vi "Run.vi"(7 "Team Index":i32, 8 "Column":i32, 9 "Row":i32, 10 "View":i32[](array[numeric]) caption="View (Team Index, -1: empty)", 11 "DNatt In":refnum<class "DNatt.lvclass">) -> (0 "Replicated":refnum<class "Square.lvclass">, 1 "Direction":T1, 2 "Action":T2, 3 "DNatt Out":refnum<class "Square.lvclass">)   [LabVIEW 2015, in "DNatt.lvclass"]
uses:
  DNatt.lvclass
  Square/Square.lvclass
  Type Defs/Action Enum.ctl
  Type Defs/Direction Enum.ctl
  DNatt.lvclass/DNatt.ctl
  Common/Position.ctl
  SubVIs/Read-Only Globals.vi
  SubVIs/Globals (private).vi
  Common/Common.lvlib
  Type Defs/SB Type Defs.lvlib
panel:
  # "NW\nN\nNE\nE\nSE\nS\nSW\nW"
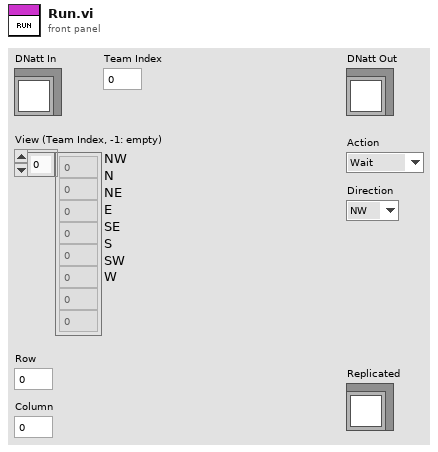
[diagram p1: front panel]
types:
  T1 = typedef "SB Type Defs.lvlib/Direction Enum.ctl" = enum16{"NW", "N", "NE", "E", "SE", "S", "SW", "W"}
  T2 = typedef "SB Type Defs.lvlib/Action Enum.ctl" = enum16{"Wait", "Move", "Attack", "Replicate"}
  T3 = typedef "Common.lvlib/Map DVR.ctl" = refnum<data-value>
  T4 = typedef "Common.lvlib/Position.ctl" = cluster{"Column":i32, "Row":i32}
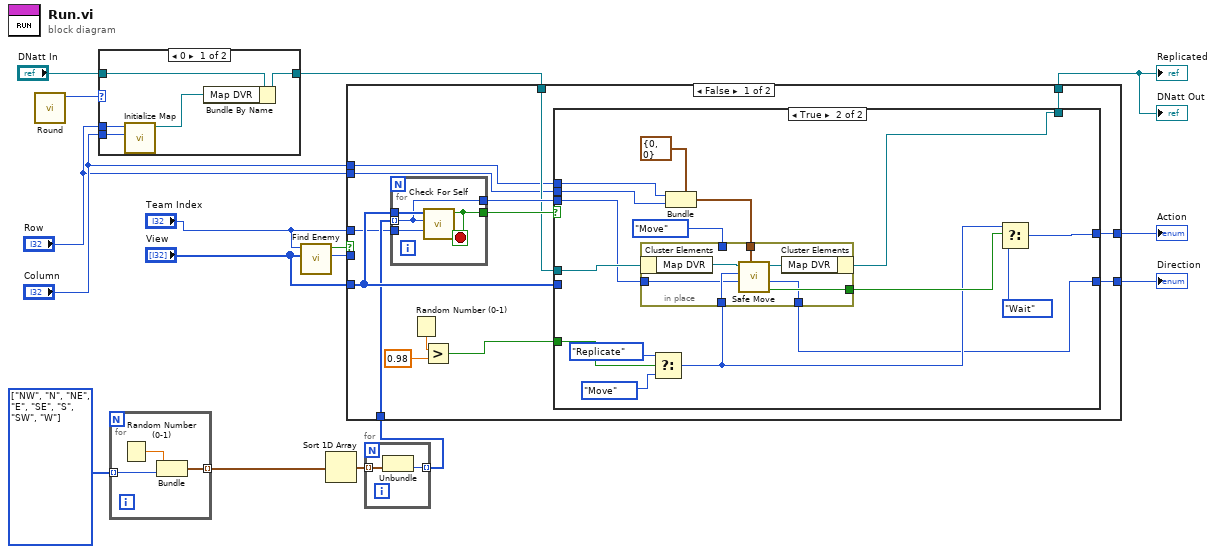
[diagram p0: block diagram]
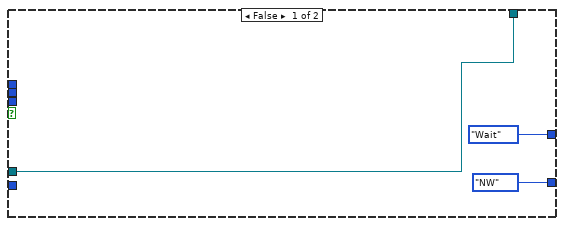
[diagram p3: hidden frame]
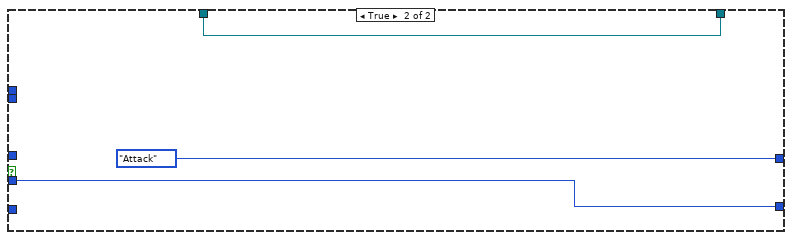
[diagram p4: hidden frame]
diagram:
  w11 = T1[] [enum."NW", enum."N", enum."NE", enum."E", enum."SE", enum."S", enum."SW", enum."W"] items=["NW", "N", "NE", "E", "SE", "S", "SW", "W"]
  n1 = call "Round.vi"() -> ("Round"=w6:i32)  [unwired: 11 in]
  n2 = case shown="0" w6 {
    tunnel: "DNatt In" -> [w19 w22]
    tunnel: [w18 w22] -> w5
    tunnel: "Row" -> [w21 _]
    tunnel: "Column" -> [w20 _]
    frame 0 {
      n3 = call "Initialize Map.vi"("Column"=w20, "Row"=w21) -> ("Map DVR"=w17:T3)  [unwired: 9 in]
      n4 = Bundle By Name(cluster=w19, "Map DVR"=w17) -> (w18:refnum<class "DNatt.lvclass">)
    }
    frame Default {
    }
  }
  n5 = for {
    tunnel: w11 -> [w24] mode=indexing
    tunnel: [w23] -> w10 mode=indexing
    n6 = Random Number (0-1)() -> (number: 0 to 1=w25:dbl)
    n7 = Bundle("number: 0 to 1"=w25, "Direction"=w24) -> (w23:cluster{"number: 0 to 1":dbl, "Direction":T1})  [unwired: 1 in]
  }
  n8 = call "Find Enemy.vi"("View"="View", "Team Index"="Team Index") -> ("Direction"=w15:T1, "Found Enemy?"=w16:bool)  [unwired: 7 in, 1 out]
  n9 = Sort 1D Array(array=w10) -> (sorted array=w9:cluster{"number: 0 to 1":dbl, "Direction":T1}[])
  n10 = for {
    tunnel: w9 -> [w27] mode=indexing
    tunnel: [w26] -> w8 mode=indexing
    n11 = Unbundle(w27) -> ("Direction"=w26:T1)  [unwired: 1 out]
  }
  n12 = case shown="False" w16 {
    tunnel: w15 -> [_ w73]
    tunnel: [w41 Action_Enum."Attack" ("Action")] -> w14
    tunnel: [w37 w73] -> w13
    tunnel: "View" -> [w40 _]
    tunnel: w8 -> [w39 _]
    tunnel: w5 -> [w32 w72]
    tunnel: [w31 w72] -> w4
    tunnel: "Column" -> [w30 _]
    tunnel: "Row" -> [w29 _]
    tunnel: "Team Index" -> [w28 _]
    frame False {
      n13 = for {
        tunnel: w40 -> [w71]
        tunnel: w39 -> [w69] mode=indexing
        tunnel: [w70] -> w38
        tunnel: [w69] -> w36
        tunnel: w28 -> [w68]
        stop <- w70 stop-if-true
        n14 = call "Check For Self.vi"("Team index"=w68, "Direction"=w69, "Map"=w71) -> ("Clear?"=w70:bool)  [unwired: 8 in]
      }
      n15 = Random Number (0-1)() -> (number: 0 to 1=w35:dbl)
      n16 = Greater?(x=w35, y=0.98) -> (0:w33:bool)
      n17 = case shown="True" w38 {
        tunnel: w33 -> [_ w53]
        tunnel: [Action_Enum."Wait" ("Action") w60] -> w41
        tunnel: w40 -> [_ _]
        tunnel: [Direction_Enum."NW" ("Direction") w45] -> w37
        tunnel: w36 -> [_ w50]
        tunnel: w32 -> [w42 w56]
        tunnel: [w42 w48] -> w31
        tunnel: w30 -> [_ w54]
        tunnel: w29 -> [_ w55]
        frame False {
        }
        frame True {
          n18 = Select(t=Action_Enum."Replicate" ("Action"), s=w53, f=Action_Enum."Move" ("Action")) -> (s? t:f=w46:T2)
          n19 = Bundle(cluster=T4 {"Column"=0, "Row"=0} ("Position in"), "Column"=w54, "Row"=w55) -> (w59:T4)
          n20 = in-place {
            in-place-border: Action_Enum."Move" ("Action") -> [_]
            in-place-border: [w65] -> w47
            in-place-border: w59 -> [w64]
            in-place-border: w46 -> [w63]
            in-place-border: w50 -> [w62]
            in-place-border: [w61] -> w45
            n21 = in-place-cluster #1(w56) -> ("Map DVR"=w67:T3)
            n22 = call "Safe Move.vi"("Position in"=w64, "Direction in"=w62, "Desired Action"=w63, "Map DVR"=w67) -> ("Accepted?"=w65:bool, "Direction"=w61:T1, "Map DVR out"=w66:T3)  [unwired: 4 in, 1 out]
            n23 = in-place-cluster #1("Map DVR"=w66) -> (w48:refnum<class "DNatt.lvclass">)
          }
          n24 = Select(t=w46, s=w47, f=Action_Enum."Wait" ("Action")) -> (s? t:f=w60:T2)
        }
      }
    }
    frame True {
    }
  }
  "DNatt Out" <- w4
  "Action" <- w14
  "Direction" <- w13
  "Replicated" <- w4
